vi "DataLog Next Capacity Power Of Two.vi"(2 "lower limit":i32, 3 "min capacity":i32) -> (0 "mask (2^N-1)":i32 format="%.0x", 1 "actual capacity (2^N)":i32)   [LabVIEW 2012]
doc: "Calculate the lowest 2^N buffer capacity and 2^N-1 buffer large enough to provide the desired capacity or lower limit (whichever is larger)."
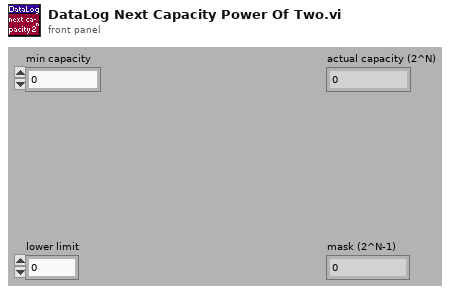
[diagram p1: front panel]
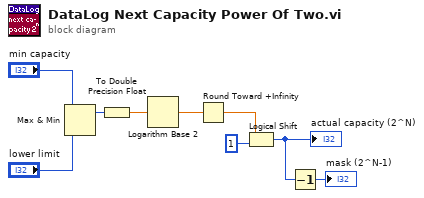
[diagram p0: block diagram]
diagram:
  n1 = Max & Min(x="min capacity", y="lower limit") -> (max(x,y)=w4:i32)  [unwired: 1 out]
  n2 = To Double Precision Float(number=w4) -> (double precision float=w3:dbl)
  n3 = Logarithm Base 2(1:w3) -> (0:w2:dbl)
  n4 = Round Toward +Infinity(x=w2) -> (ceil(x): smallest int >= x=w1:dbl)
  n5 = Logical Shift(y=w1, x=1) -> (x << y=w6:i32)
  "actual capacity (2^N)" <- w6
  n6 = Decrement(x=w6) -> (x-1=→"mask (2^N-1)":i32)
